vi "Execute.vi"(6 "commandTimeout":i32=-1, 7 "CommandType":i32(ring)=-1 items=["Text"=1, "StoredProcedure"=4, "TableDirect"=512], 8 "error in (no error)":errorcluster, 9 "DynamicParameters":refnum<class "DynamicParameters.lvclass">, 10 "sql":string, 11 "SqlMapper in":refnum<class "DapperMapper.lvclass">) -> (0 "error out":errorcluster, 2 "affectedRows":i32, 3 "SqlMapper out":refnum<class "DapperMapper.lvclass">)   [LabVIEW 2020, in "ORM_Dapper.lvlib" / "DapperMapper.lvclass"]
uses:
  DapperMapper.lvclass
  C:/Program Files/National Instruments/LabVIEW 2024/vi.lib/Viviota/shared/ORM.lvlibp/ORM/SqlMapper/SqlMapper.lvclass
  <vilib>/Viviota/shared/ORM.lvlibp/ORM/DynamicParameters/DynamicParameters.lvclass
  DapperParameters/DapperParameters.lvclass
  <vilib>/Viviota/shared/ORM_DBC_dotNet.lvlibp/dbcDotNet/ORM_DBC_dotNet.lvclass
  DapperParameters/DapperParameters.lvclass/DapperParameters.ctl
  <vilib>/Viviota/shared/ORM.lvlibp/ORM/SqlMapper/Read DbConnection.vi
  <vilib>/Viviota/shared/ORM_DBC_dotNet.lvlibp/dbcDotNet/Read connection.vi
  <vilib>/Viviota/shared/ORM_DBC_dotNet.lvlibp/dbcDotNet/Read transaction.vi
  C:/Viviota/Projects/R&D/__OpenSource/VIV_ORM/libraries/dapper/Dapper.dll
  libraries/dapper/Dapper.dll
  <vilib>/Viviota/shared/ORM.lvlibp/ORM/DbConnection/DbConnection.lvclass
  System.Data
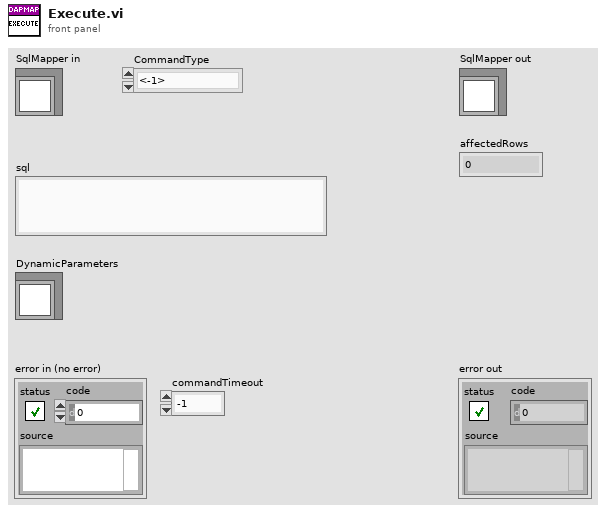
[diagram p1: front panel]
types:
  T1 = typedef "ORM_Dapper.lvlib/dapper_sqlmapper_ref.ctl" = refnum<k24>
  T2 = typedef "ORM_Dapper.lvlib/dapper_dynamicparameters_ref.ctl" = refnum<k24>
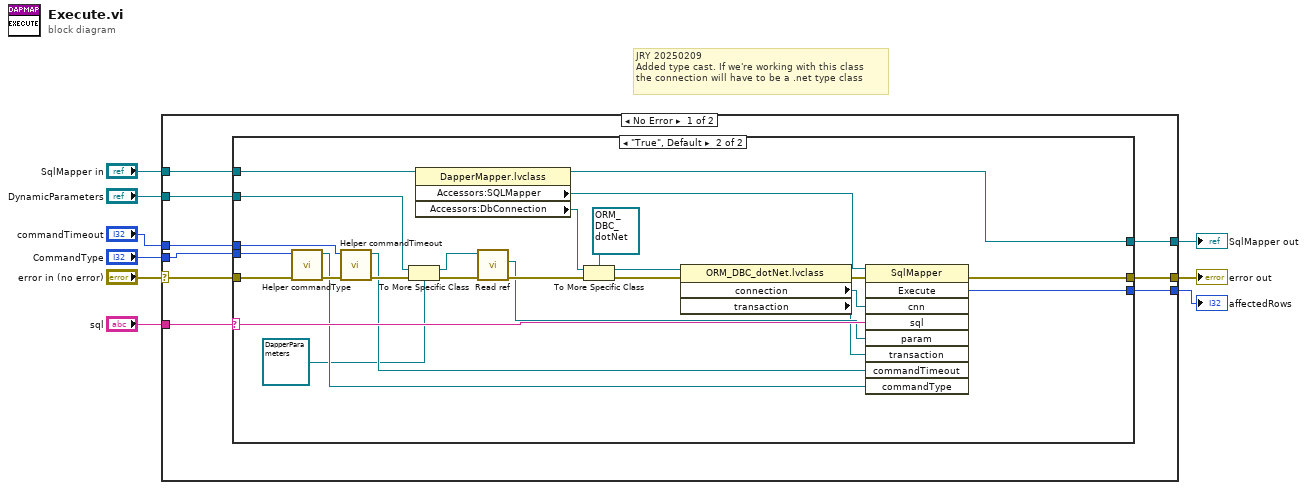
[diagram p0: block diagram]
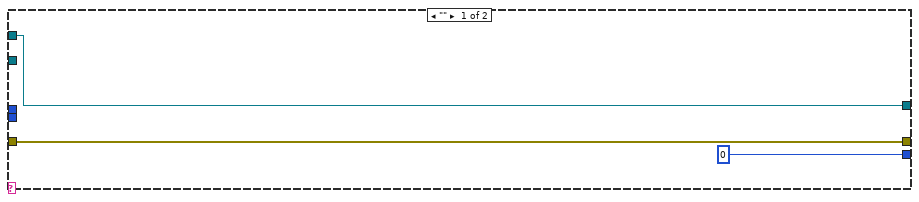
[diagram p2: hidden frame]
diagram:
  # "JRY 20250209\nAdded type cast. If we're working with this class\nthe connection will have to be a .net type class"
  n1 = case shown="No Error" "error in (no error)" {
    selector: "error in (no error)" -> [w13 w49]
    tunnel: [w16 w49] -> w8
    tunnel: [w11 w48] -> w6
    tunnel: "SqlMapper in" -> [w12 w48]
    tunnel: "sql" -> [w18 _]
    tunnel: "CommandType" -> [w17 _]
    tunnel: "DynamicParameters" -> [w14 _]
    tunnel: [w15 _] -> w2
    tunnel: "commandTimeout" -> [w10 _]
    frame No Error {
      n2 = case shown="\"True\", Default" w18 {
        selector: w18 -> [_ w47]
        tunnel: w17 -> [_ w46]
        tunnel: [w20 w45] -> w16
        tunnel: [0 ("Execute") w44] -> w15
        tunnel: w14 -> [_ w28]
        tunnel: w13 -> [w20 w42]
        tunnel: w12 -> [w21 w41]
        tunnel: [w21 w31] -> w11
        tunnel: w10 -> [_ w32]
        frame "" {
        }
        frame "True", Default {
          n3 = call "Helper commandType.vi"("error in (no error)"=w42, "CommandType"=w46) -> ("error out"=w43:errorcluster, ".NET Refnum out"=w35:refnum<k24>)  [unwired: 8 in]
          n4 = call "Helper commandTimeout.vi"("error in (no error)"=w43, "commandTimeout in"=w32) -> ("error out"=w40:errorcluster, ".NET Refnum out"=w36:refnum<k24>)  [unwired: 8 in]
          n5 = To More Specific Class(target class=refnum<class "DapperParameters.lvclass"> refnum ("Dapper.lvlib:DynamicParameters"), reference=w28, error in=w40) -> (specific class reference=w27:refnum<class "DapperParameters.lvclass">, error out=w29:errorcluster)
          n6 = property class="DapperMapper.lvclass"(reference=w41) -> (reference out=w31:refnum<class "DapperMapper.lvclass">, "Accessors:SQLMapper"=w30:T1, "Accessors:DbConnection"=w24:refnum<class "DbConnection.lvclass">)  [unwired: 1 in, 1 out]
          n7 = call "Read ref.vi"("error in (no error)"=w29, "DynamicParameters in"=w27) -> ("error out"=w39:errorcluster, "ref"=w37:T2)  [unwired: 7 in, 1 out]
          n8 = To More Specific Class(target class=refnum<class "ORM_DBC_dotNet.lvclass"> refnum ("ORM_DBC_dotNet.lvlibp:ORM_DBC_dotNet.lvclass"), reference=w24, error in=w39) -> (specific class reference=w23:refnum<class "ORM_DBC_dotNet.lvclass">, error out=w25:errorcluster)
          n9 = property class="ORM_DBC_dotNet.lvclass"(reference=w23, error in=w25) -> (error out=w38:errorcluster, "connection"=w33:refnum<k24>, "transaction"=w34:refnum<k24>)  [unwired: 1 out]
          n10 = invoke class="SqlMapper" method="Execute"(reference=w30, error in=w38, "cnn"=w33, "sql"=w47, "param"=w37, "transaction"=w34, "commandTimeout"=w36, "commandType"=w35) -> (error out=w45:errorcluster, "Execute"=w44:i32)  [unwired: 1 in, 7 out]
        }
      }
    }
    frame Error {
    }
  }
  "error out" <- w8
  "SqlMapper out" <- w6
  "affectedRows" <- w2
